vi "Normalize Path.vi"(11 "Image Directory":path) -> (0 "Filenames":string[](array[string]), 3 "Path":path)   [LabVIEW 2015]
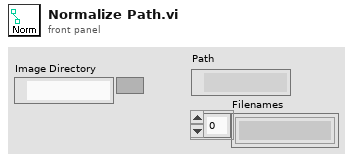
[diagram p1: front panel]
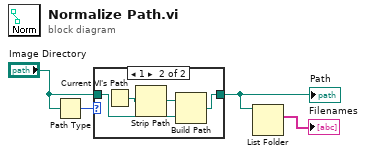
[diagram p0: block diagram]
diagram:
  n1 = Path Type(1:"Image Directory") -> (0:w3:i16)
  n2 = case shown="1" w3 {
    tunnel: "Image Directory" -> [w5 w9]
    tunnel: [w5 w6] -> w2
    frame 0, Default {
    }
    frame 1 {
      n3 = Current VI's Path() -> (path=w8:path)
      n4 = Strip Path(path=w8) -> (stripped path=w7:path)  [unwired: 1 out]
      n5 = Build Path(base path=w7, name or relative path=w9) -> (appended path=w6:path)
    }
  }
  "Path" <- w2
  n6 = List Folder(path=w2) -> (filenames=→"Filenames":string[])  [unwired: 3 in, 3 out]
